vi "Execute Script.vi"(0 "Scripts Dir":path, 5 "uids":string[](array[string]), 7 "QD Plugins Dir":path, 9 "Arguments":string[](array[string]), 11 "error in (no error)":errorcluster, 12 "VI Refnum":refnum<vi>, 13 "Focus":enum8{"FP", "BD"}(ring), 14 "Shift?":bool) -> (15 "error out":errorcluster)   [LabVIEW 2019, in "Script.lvlib"]
doc: "Execute a Script VI from the uids formatted as: UID=VI:SHORTCUT\n\nCreated By: Ryan Pacini"
uses:
  Script.lvlib
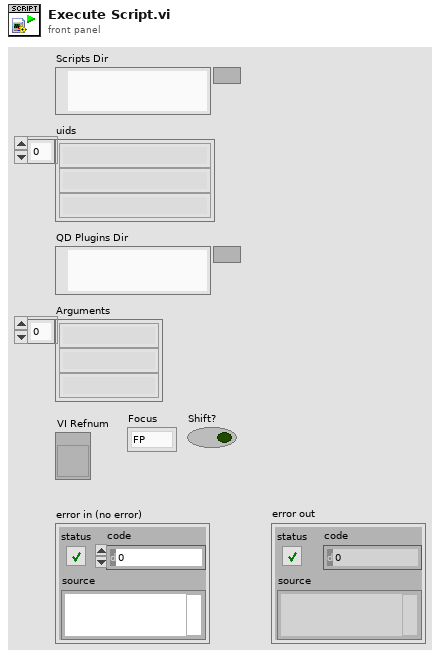
[diagram p1: front panel]
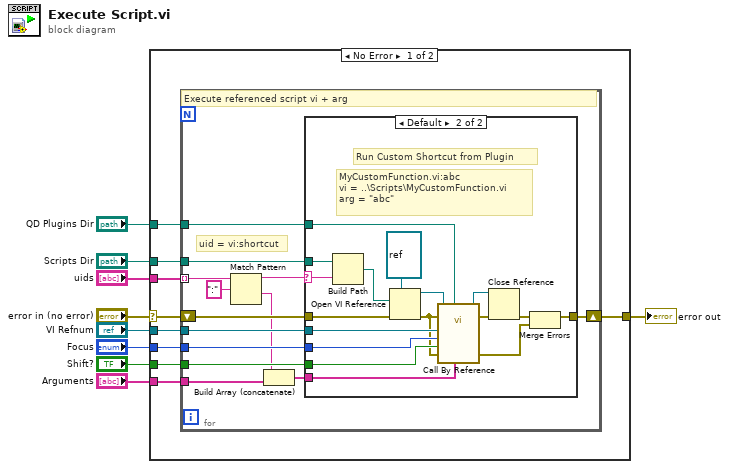
[diagram p0: block diagram]
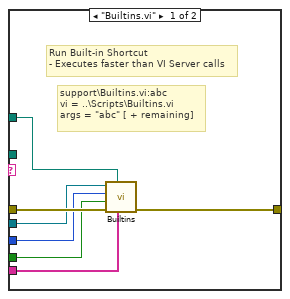
[diagram p2: hidden frame]
diagram:
  n1 = case shown="No Error" "error in (no error)" {
    selector: "error in (no error)" -> [w11 w56]
    tunnel: "QD Plugins Dir" -> [w18 _]
    tunnel: "Arguments" -> [w17 _]
    tunnel: "Scripts Dir" -> [w16 _]
    tunnel: [w15 w56] -> w1
    tunnel: "Shift?" -> [w14 _]
    tunnel: "Focus" -> [w13 _]
    tunnel: "VI Refnum" -> [w12 _]
    tunnel: "uids" -> [w10 _]
    frame No Error {
      n2 = for {
        tunnel: w10 -> [w25] mode=indexing
        tunnel: w12 -> [w30]
        tunnel: w13 -> [w29]
        tunnel: w14 -> [w28]
        shift-right: [w27] -> w15
        shift-left: w11 -> [w31]
        tunnel: w16 -> [w22]
        tunnel: w17 -> [w21]
        tunnel: w18 -> [w19]
        # "uid = vi:shortcut"
        # "Execute referenced script vi + arg"
        n3 = Match Pattern(string=w25, regular expression=":") -> (before substring=w23:string, after substring=w26:string)  [unwired: 1 in, 2 out]
        n4 = Build Array (concatenate)(w26, w21) -> (w20:string[])
        n5 = case shown="Default" w23 {
          selector: w23 -> [_ w43]
          tunnel: w31 -> [w38 w55]
          tunnel: w30 -> [w37 w52]
          tunnel: w29 -> [w36 w51]
          tunnel: w28 -> [w35 w50]
          tunnel: [w34 w45] -> w27
          tunnel: w22 -> [_ w42]
          tunnel: w20 -> [w33 w40]
          tunnel: w19 -> [w32 w39]
          frame "Builtins.vi" {
            # "support\\Builtins.vi:abc\nvi = ..\\Scripts\\Builtins.vi\nargs = \"abc\" [ + remaining]"
            # "Run Built-in Shortcut\n- Executes faster than VI Server calls"
            n6 = call "Builtins.vi"("args"=w33, "QD Plugins Dir"=w32, "error in (no error)"=w38, "Shift?"=w35, "Focus"=w36, "VI Refnum"=w37) -> ("error out"=w34:errorcluster)  [unwired: 5 in]
          }
          frame Default {
            # "Run Custom Shortcut from Plugin"
            # "MyCustomFunction.vi:abc\nvi = ..\\Scripts\\MyCustomFunction.vi\narg = \"abc\""
            n7 = Build Path(base path=w42, name or relative path=w43) -> (appended path=w41:path)
            n8 = Open VI Reference(type specifier VI Refnum (for type only)=refnum<vi> refnum, vi path=w41, error in (no error)=w55) -> (vi reference=w53:refnum<vi>, error out=w49:errorcluster)  [unwired: 3 in]
            n9 = call-by-ref "?"(reference=w53, error in=w49, "args"=w40, "QD Plugins Dir"=w39, 8:"error in (no error)"=w49, "Shift?"=w50, "Focus"=w51, "VI Refnum"=w52) -> (reference out=w47:refnum<vi>, error out=w48:errorcluster, 0:"error out"=w44:errorcluster)  [unwired: 5 in]
            n10 = Close Reference(reference=w47, error in (no error)=w48) -> (error out=w46:errorcluster)
            n11 = Merge Errors(w46, w44) -> (w45:errorcluster)
          }
        }
      }
    }
    frame Error {
    }
  }
  "error out" <- w1
